vi "Modifiers Down.vi"(7 "Delay":i32, 8 "error in (no error)":errorcluster, 9 "Shift?":bool, 10 "Alt?":bool, 11 "Ctrl?":bool) -> (0 "error out":errorcluster)   [LabVIEW 2020, in "MacroAssert.lvlib"]
uses:
  MacroAssert.lvlib
  eeabe754-8c5a-4123-a515-6e4897587338.vi
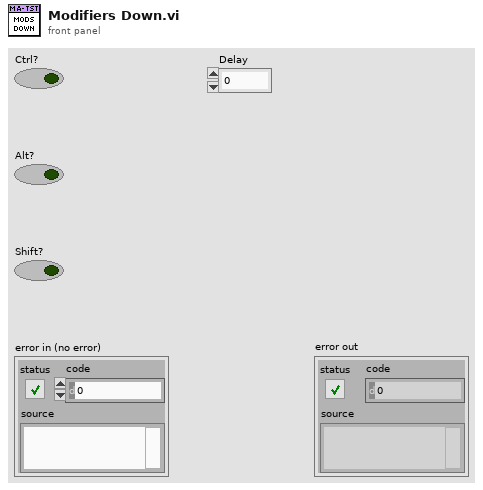
[diagram p1: front panel]
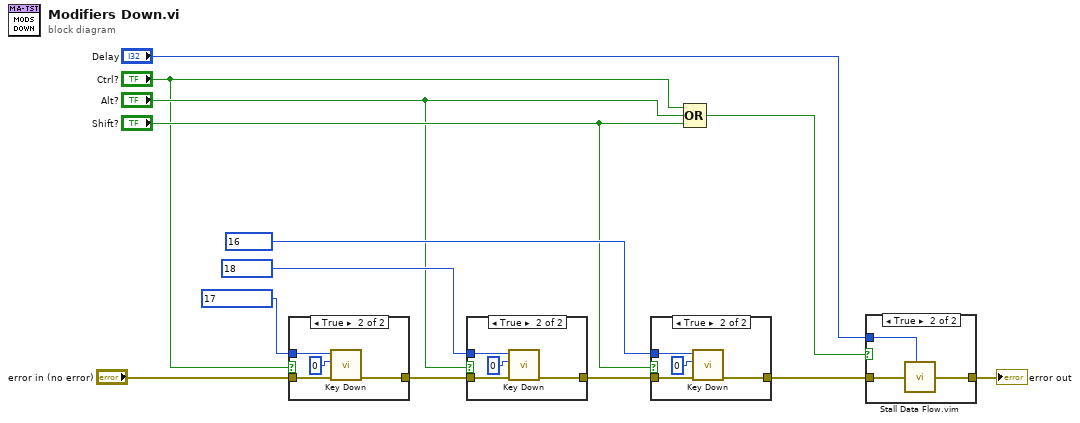
[diagram p0: block diagram]
diagram:
  n1 = case shown="True" "Ctrl?" {
    tunnel: "error in (no error)" -> [w14 w18]
    tunnel: [w14 w17] -> w12
    tunnel: u8 17 ("Virtual Key") -> [_ w16]
    frame False {
    }
    frame True {
      n2 = call "Key Down.vi"("error in (no error)"=w18, "delay in ms (80)"=u32 0, "Virtual Key"=w16) -> ("error out"=w17:errorcluster)  [unwired: 8 in]
    }
  }
  n3 = case shown="True" "Alt?" {
    tunnel: w12 -> [w19 w23]
    tunnel: [w19 w22] -> w11
    tunnel: u8 18 ("Virtual Key") -> [_ w21]
    frame False {
    }
    frame True {
      n4 = call "Key Down.vi"("error in (no error)"=w23, "delay in ms (80)"=u32 0, "Virtual Key"=w21) -> ("error out"=w22:errorcluster)  [unwired: 8 in]
    }
  }
  n5 = case shown="True" "Shift?" {
    tunnel: w11 -> [w24 w28]
    tunnel: [w24 w27] -> w7
    tunnel: u8 16 ("Virtual Key") -> [_ w26]
    frame False {
    }
    frame True {
      n6 = call "Key Down.vi"("error in (no error)"=w28, "delay in ms (80)"=u32 0, "Virtual Key"=w26) -> ("error out"=w27:errorcluster)  [unwired: 8 in]
    }
  }
  n7 = Compound Arithmetic op=OR("Ctrl?", "Alt?", "Shift?") -> (w2:bool)
  n8 = case shown="True" w2 {
    tunnel: w7 -> [w29 w32]
    tunnel: [w29 w31] -> w6
    tunnel: "Delay" -> [_ w30]
    frame False {
    }
    frame True {
      n9 = call "Stall Data Flow.vim"("value in"=w32, "milliseconds to wait"=w30) -> ("value out"=w31:errorcluster)  [unwired: 1 out]
    }
  }
  "error out" <- w6
